vi "type-k-conversion.vi"(8 "error in (no error)":errorcluster, 11 "object in":refnum<class "Sensor-Class.lvclass">) -> (0 "error out":errorcluster, 3 "object out":refnum<class "Sensor-Class.lvclass">)   [LabVIEW 2016, in "Sensor-Class.lvclass"]
doc: "thermocouples Type K"
uses:
  Sensor-Class.lvclass
  Sensor-Class.lvclass/Sensor-Class.ctl
panel:
  # "Conversion modbus to Type K"
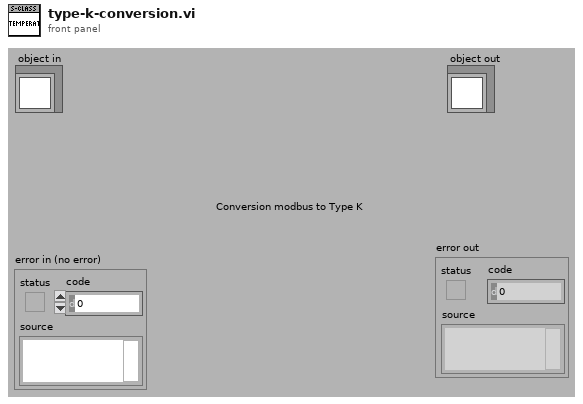
[diagram p1: front panel]
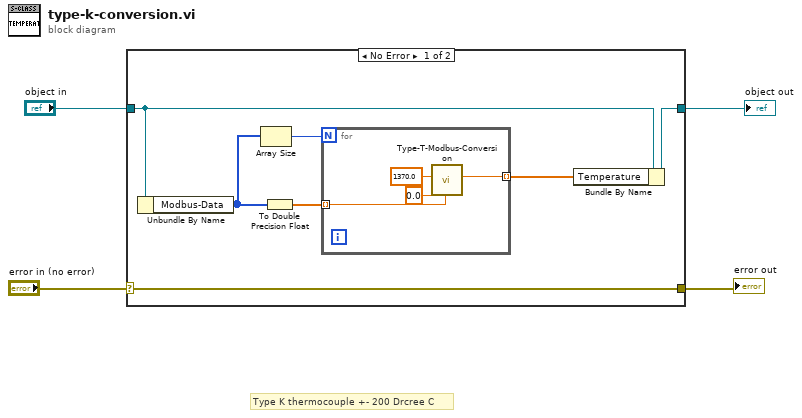
[diagram p0: block diagram]
diagram:
  # "Type K thermocouple +- 200 Drcree C"
  n1 = case shown="No Error" "error in (no error)" {
    selector: "error in (no error)" -> [w6 w17]
    tunnel: [w6 w17] -> w3
    tunnel: [w11 w16] -> w1
    tunnel: "object in" -> [w10 w16]
    frame No Error {
      n2 = Unbundle By Name(w10) -> ("Modbus-Data"=w8:u16[])
      n3 = Array Size(array=w8) -> (size(s)=w9:i32)
      n4 = To Double Precision Float(number=w8) -> (double precision float=w5:dbl[])
      n5 = for {
        N: w9 -> [_]
        tunnel: w5 -> [w15] mode=indexing
        tunnel: [w14] -> w7 mode=indexing
        n6 = call "Type-T-Modbus-Conversion.vi"("Reg"=w15, "Scale Min range"=0.0, "Scale Max Range"=1370.0) -> ("output"=w14:dbl)  [unwired: 7 in, 1 out]
      }
      n7 = Bundle By Name(cluster=w10, "Temperature"=w7) -> (w11:refnum<class "Sensor-Class.lvclass">)
    }
    frame Error {
    }
  }
  "error out" <- w3
  "object out" <- w1
